vi "AssetMgrExportAssetTemplateResponse_Name.vi"() -> (1 "MessageName":string)   [LabVIEW 2017]
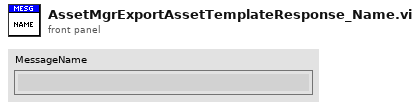
[diagram p1: front panel]
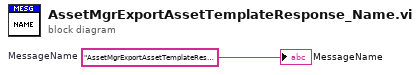
[diagram p0: block diagram]
diagram:
  w1 = "AssetMgrExportAssetTemplateResponse"  # MessageName
  "MessageName" <- w1
